vi "Distance.vi"(1 "Feet":dbl) -> (0 "Distance":dbl)   [LabVIEW 2014]
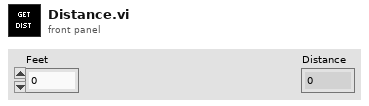
[diagram p1: front panel]
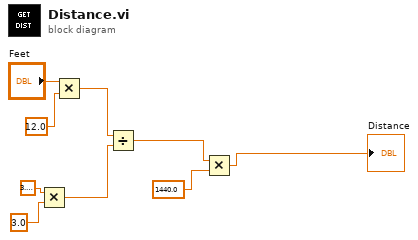
[diagram p0: block diagram]
diagram:
  n1 = Multiply(x=3.141592653589793, y=3.0) -> (x*y=w2:dbl)
  n2 = Multiply(x="Feet", y=12.0) -> (x*y=w3:dbl)
  n3 = Divide(x=w3, y=w2) -> (x/y=w1:dbl)
  n4 = Multiply(x=w1, y=1440.0) -> (x*y=→"Distance":dbl)
